vi "initLoopConfig.vi"(8 "error in (no error)":errorcluster, 10 "configDirectoryPathWindows":path, 11 "LoopConfig in":refnum<class "LoopConfig.lvclass">) -> (0 "error out":errorcluster, 3 "LoopConfig out":refnum<class "LoopConfig.lvclass">)   [LabVIEW 2013, in "ComponentData.lvlib" / "LoopConfig.lvclass"]
uses:
  <userlib>/Common/Component/common_application/RT/ComponentData/ConfigurationHandler/LoopConfig/LoopConfig.lvclass
  <userlib>/Common/Component/common_application/MyComputer/ComponentConfiguration/ComponentConfigurationTypedefs/loopConfig.ctl
  <userlib>/Common/Component/common_application/RT/ComponentData/ConfigurationHandler/LoopConfig/LoopConfig.lvclass/LoopConfig.ctl
  <vilib>/Utility/xml.llb/Read From XML File(string).vi
  <userlib>/Common/Component/common_application/MyComputer/ComponentConfiguration.lvlib
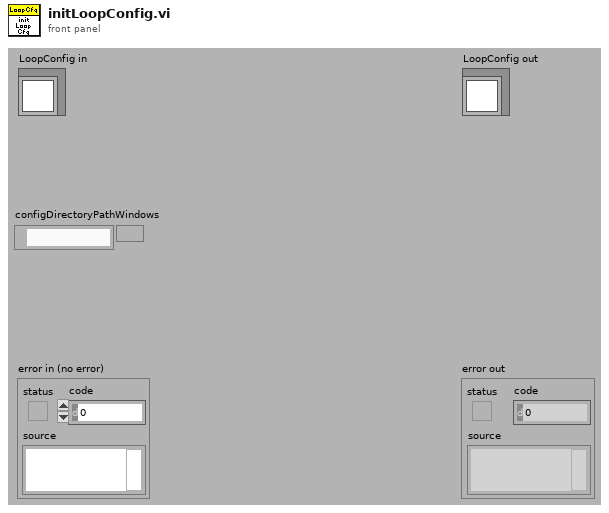
[diagram p1: front panel]
types:
  T1 = typedef "ComponentConfiguration.lvlib/loopConfig.ctl" = cluster{"hostLoopPeriod_s":dbl, "hostLoopPeriodAllowedJitter_percent":dbl}
  T2 = enum32{"invalid OS target", "Mac OS", "Windows 3.1", "Windows 95/NT", "Solaris 1", "Solaris 2", "HP-UX", "PowerMAX", "Linux", "Irix", "Rhapsody", "BeOS", "AIX", "OSF1", "VxWorks", "PharLap", "Carbon", "RTX", "Windows x64", "Linux x64"}
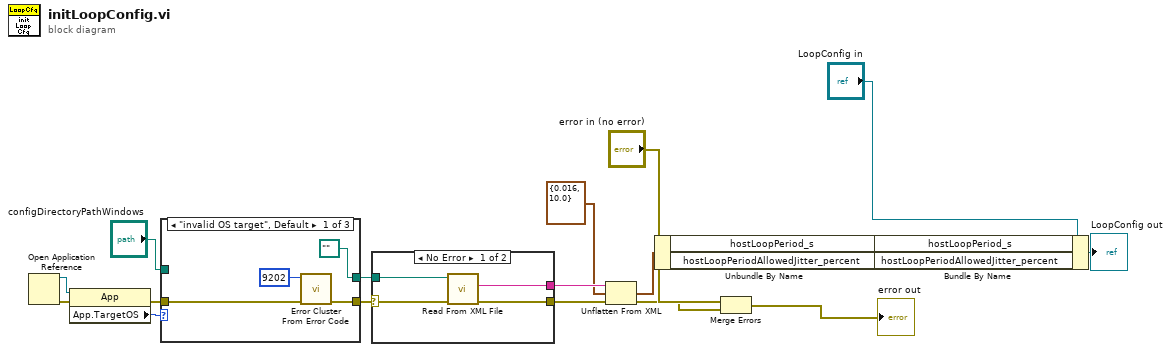
[diagram p0: block diagram]
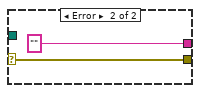
[diagram p2: hidden frame]
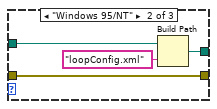
[diagram p3: hidden frame]
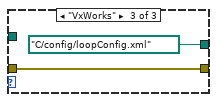
[diagram p4: hidden frame]
diagram:
  n1 = Open Application Reference() -> (0:w7:errorcluster, 3:w10:refnum<vi>)  [unwired: 4 in]
  n2 = property class="App"(reference=w10, error in=w7) -> (error out=w6:errorcluster, "App.TargetOS"=w9:T2)  [unwired: 1 out]
  n3 = case shown="\"invalid OS target\", Default" w9 {
    tunnel: [path "" ("configuration file path") w26 path "C:/config/loopConfig.xml" ("configuration file path")] -> w8
    tunnel: w6 -> [w20 w25 w27]
    tunnel: [w19 w25 w27] -> w5
    tunnel: "configDirectoryPathWindows" -> [_ w23 _]
    frame "invalid OS target", Default {
      n4 = call <vilib>:"Error Cluster From Error Code.vi"("error in (no error)"=w20, "error code (0)"=9202) -> ("error out"=w19:errorcluster)  [unwired: 7 in]
    }
    frame "Windows 95/NT" {
      n5 = Build Path(base path=w23, name or relative path="loopConfig.xml") -> (appended path=w26:path)
    }
    frame "VxWorks" {
    }
  }
  n6 = case shown="No Error" w5 {
    selector: w5 -> [w29 w33]
    tunnel: w8 -> [w32 _]
    tunnel: [w31 "" ("XML Elements")] -> w16
    tunnel: [w30 w33] -> w11
    frame No Error {
      n7 = call-poly <vilib>:"Read From XML File.vi"("error in (no error)"=w29, "XML File Path"=w32) -> ("error out"=w30:errorcluster, "XML Elements"=w31:string)  [unwired: 7 in, 1 out]
    }
    frame Error {
    }
  }
  n8 = Unflatten From XML(xml string=w16, type=T1 {"hostLoopPeriod_s"=0.016, "hostLoopPeriodAllowedJitter_percent"=10.0} ("loopConfig"), error in (no error)=w11) -> (value=w14:T1, error out=w2:errorcluster)
  n9 = Unbundle By Name(w14) -> ("hostLoopPeriod_s"=w13:dbl, "hostLoopPeriodAllowedJitter_percent"=w12:dbl)
  n10 = Merge Errors("error in (no error)", w2) -> (→"error out":errorcluster)
  n11 = Bundle By Name(cluster="LoopConfig in", "hostLoopPeriod_s"=w13, "hostLoopPeriodAllowedJitter_percent"=w12) -> (→"LoopConfig out":refnum<class "LoopConfig.lvclass">)
